vi "FGV_FOV strings and values.vi"(8 "error in (no error)":errorcluster, 11 "FOV control Strings And Values":T1=[{"String"="175 µm", "Value"=4.35}, {"String"="235 µm", "Value"=5.6}, {"String"="350 µm", "Value"=8.7}]) -> (0 "error out":errorcluster, 3 "FOV control Strings And Values []":T1)   [LabVIEW 2020]
uses:
  <vilib>/Utility/miscctls.llb/LVStringsAndValuesArrayTypeDef_SGL.ctl
panel:
  # "SUB-ROUTINE"
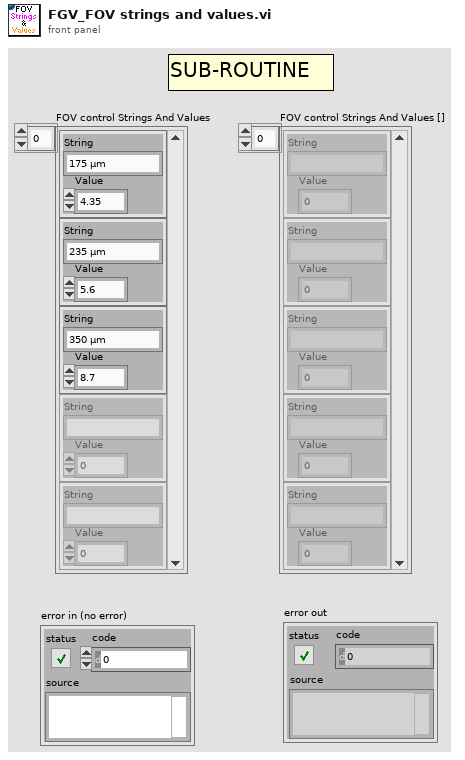
[diagram p1: front panel]
types:
  T1 = typedef "LVStringsAndValuesArrayTypeDef_SGL.ctl" = cluster{"String":string, "Value":sgl}[]
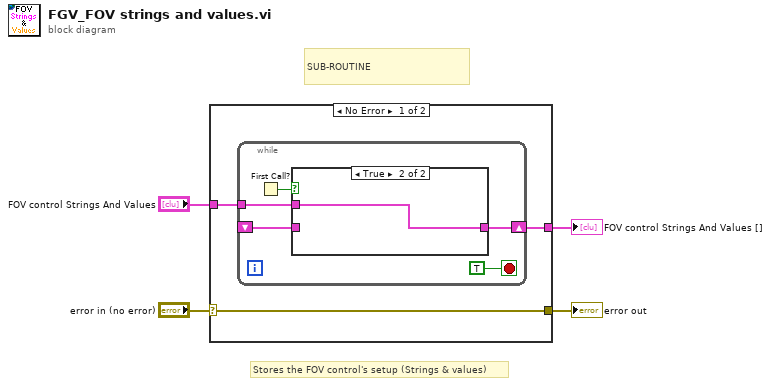
[diagram p0: block diagram]
diagram:
  # "Stores the FOV control's setup (Strings & values)"
  # "SUB-ROUTINE"
  n1 = case shown="No Error" "error in (no error)" {
    selector: "error in (no error)" -> [w5 w16]
    tunnel: [w7 w15] -> w4
    tunnel: "FOV control Strings And Values" -> [w6 w15]
    tunnel: [w5 w16] -> w1
    frame No Error {
      n2 = while {
        shift-right: [w11] -> w7
        shift-left: _ -> [w9]
        tunnel: w6 -> [w8]
        stop <- TRUE stop-if-true
        n3 = First Call?() -> (First Call?: T/F=w10:bool)
        n4 = case shown="True" w10 {
          tunnel: [w13 w14] -> w11
          tunnel: w9 -> [w13 _]
          tunnel: w8 -> [_ w14]
          frame False {
          }
          frame True {
          }
        }
      }
    }
    frame Error {
    }
  }
  "FOV control Strings And Values []" <- w4
  "error out" <- w1
